vi "destroy.vi"(8 "error in (no error)":errorcluster, 11 "librarian_sm in":refnum<class "librarian.lvclass">) -> (0 "error out":errorcluster, 3 "librarian_sm out":refnum<class "librarian.lvclass">)   [LabVIEW 2020, in "librarian.lvclass"]
uses:
  librarian.lvclass
  librarian.lvclass/librarian.ctl
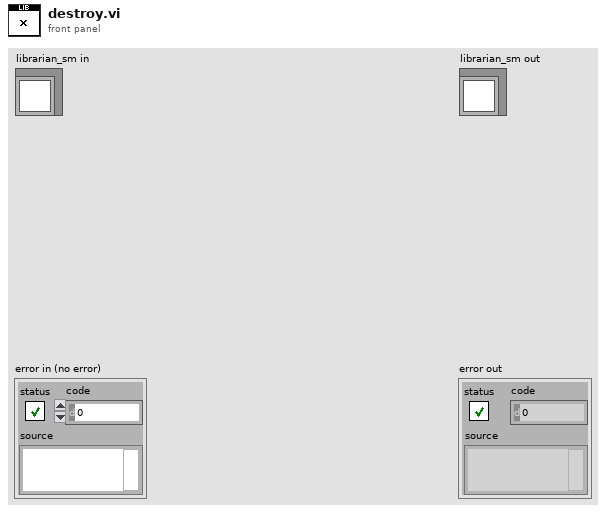
[diagram p1: front panel]
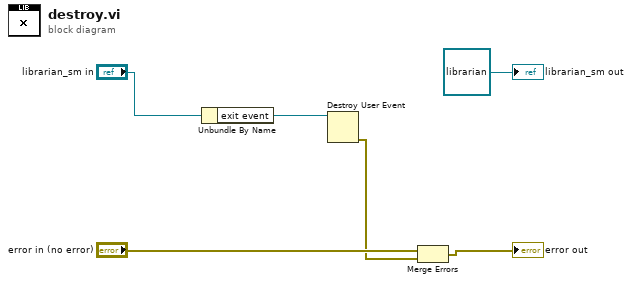
[diagram p0: block diagram]
diagram:
  n1 = Unbundle By Name("librarian_sm in") -> ("exit event"=w5:refnum<user-event>)
  n2 = Destroy User Event(user event=w5) -> (error out=w2:errorcluster)  [unwired: 1 in]
  n3 = Merge Errors("error in (no error)", w2) -> (→"error out":errorcluster)
  "librarian_sm out" <- refnum<class "librarian.lvclass"> refnum ("librarian_sm out")
